vi "main.vi"() -> ()   [LabVIEW 2023]
uses:
  cntr/Traffic_Light.ctl
panel:
  in  "Enum":enum16{"init", "gr_rt", "gr_bl", "ge", "rt_ge"}(ring)
  out "traffic light 2_2":T1
  out "traffic light 2_1":T1
  out "traffic light 1_2":T1
  out "traffic light 1_1":T1
  in  "?":T2
  in  "?":bool
  in  "Time Inputs":T3={"Green to Red"=1.0, "Yellow"=1.0, "Green blinks time"=0.5, "Blinks number"=1.0} {"Blinks number" min=1.0 max=10.0 step=1.0; "Green blinks time" min=0.5 max=2.0 step=0.5; "Yellow" min=1.0 max=10.0 step=0.5; "Green to Red" min=1.0 max=10.0 step=0.5}
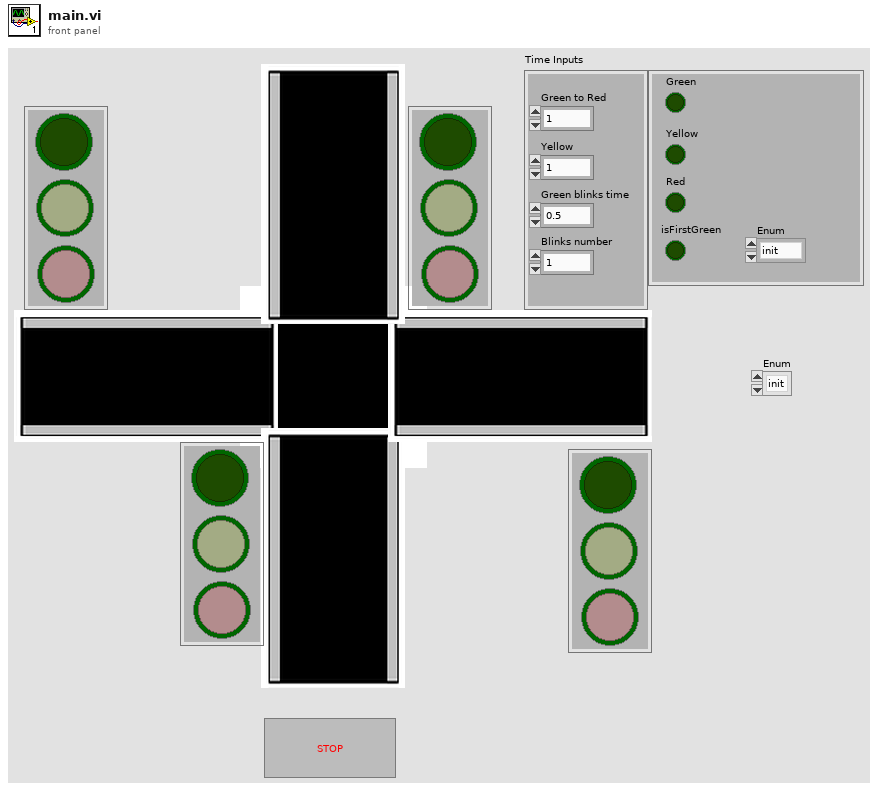
[diagram p1: front panel]
types:
  T1 = typedef "Traffic_Light.ctl" = cluster{"green":bool, "yellow":bool, "red":bool}
  T2 = cluster{"Green":bool, "Yellow":bool, "Red":bool, "isFirstGreen":bool, "Enum":enum16{"init", "gr_rt", "gr_bl", "ge", "rt_ge"}}
  T3 = cluster{"Green to Red":dbl, "Yellow":dbl, "Green blinks time":dbl, "Blinks number":dbl}
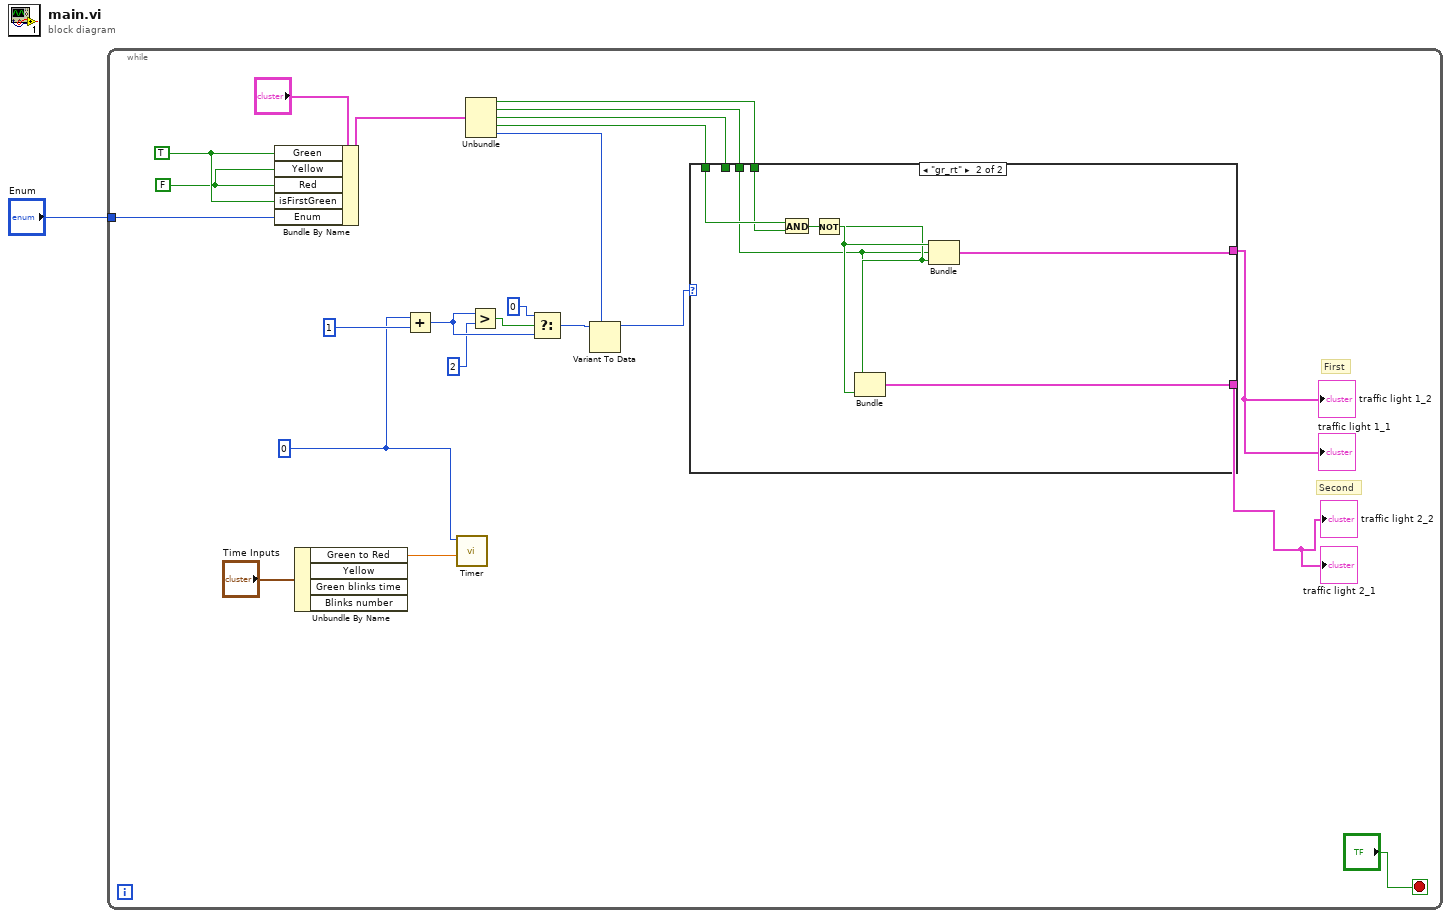
[diagram p0: block diagram]
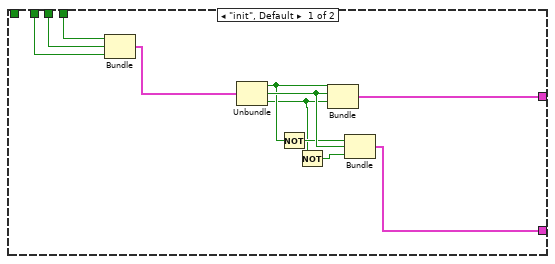
[diagram p2: hidden frame]
diagram:
  n1 = while {
    tunnel: "Enum" -> [w5]
    stop <- "?" stop-if-true
    w8 = 0
    w16 = FALSE
    w17 = TRUE
    # "Second"
    # "First"
    n2 = Bundle By Name(cluster="?", "Green"=w17, "Yellow"=w16, "Red"=w16, "isFirstGreen"=w17, "Enum"=w5) -> (w18:T2)
    n3 = Unbundle By Name("Time Inputs") -> ("Green to Red"=w20:dbl)  [unwired: 3 out]
    n4 = Add(x=w8, y=1) -> (x+y=w7:i32)
    n5 = call "Timer.vi"("Delay"=w20, "Action"=w8) -> ()  [unwired: 8 in, 2 out]
    n6 = Unbundle(w18) -> ("Green"=w11:bool, "Yellow"=w10:bool, "Red"=w9:bool, "isFirstGreen"=w12:bool, "Enum"=w4:enum16{"init", "gr_rt", "gr_bl", "ge", "rt_ge"})
    n7 = Greater?(x=w7, y=2) -> (0:w15:bool)
    n8 = Select(t=0, s=w15, f=w7) -> (s? t:f=w3:i32)
    n9 = Variant To Data(type=w4, Variant=w3) -> (data=w2:enum16{"init", "gr_rt", "gr_bl", "ge", "rt_ge"})  [unwired: 1 in, 1 out]
    n10 = case shown="\"gr_rt\"" w2 {
      tunnel: [w34 w42] -> w22
      tunnel: [w29 w41] -> w21
      tunnel: w12 -> [_ w40]
      tunnel: w11 -> [w28 w39]
      tunnel: w10 -> [w27 w36]
      tunnel: w9 -> [w26 _]
      frame "init", Default {
        n11 = Bundle("Green"=w28, "Yellow"=w27, "Red"=w26) -> (w25:cluster{"Green":bool, "Yellow":bool, "Red":bool})  [unwired: 1 in]
        n12 = Unbundle(w25) -> ("Green"=w33:bool, "Yellow"=w35:bool, "Red"=w31:bool)
        n13 = Not(x=w33) -> (.not. x?=w32:bool)
        n14 = Not(x=w31) -> (.not. x?=w30:bool)
        n15 = Bundle("Green"=w33, "Yellow"=w35, "Red"=w31) -> (w34:cluster{"Green":bool, "Yellow":bool, "Red":bool})  [unwired: 1 in]
        n16 = Bundle(w32, "Yellow"=w35, w30) -> (w29:cluster{bool, "Yellow":bool, bool})  [unwired: 1 in]
      }
      frame "gr_rt" {
        n17 = And(x=w40, y=w39) -> (x .and. y?=w38:bool)
        n18 = Not(x=w38) -> (.not. x?=w37:bool)
        n19 = Bundle(w37, "Yellow"=w36, w38) -> (w41:cluster{bool, "Yellow":bool, bool})  [unwired: 1 in]
        n20 = Bundle(w38, "Yellow"=w36, w37) -> (w42:cluster{bool, "Yellow":bool, bool})  [unwired: 1 in]
      }
    }
    "traffic light 1_2" <- w22
    "traffic light 1_1" <- w22
    "traffic light 2_1" <- w21
    "traffic light 2_2" <- w21
  }
